vi "emi_Set Time offset.vi"(7 "Offset in":dbl, 11 "error in (no error)":errorcluster) -> (15 "error out":errorcluster)   [LabVIEW 2010]
doc: "Sets the get time with error and offset offset. Does not set teh clock, and does not store the time on disk.\n\nOn error, asume that the offset is wrong. Do nothing"
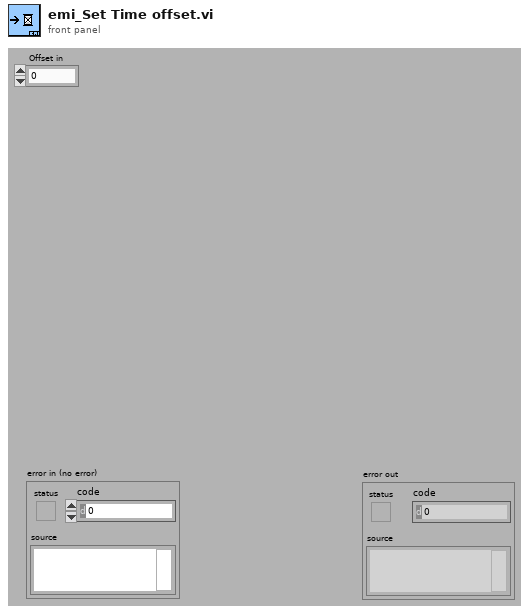
[diagram p1: front panel]
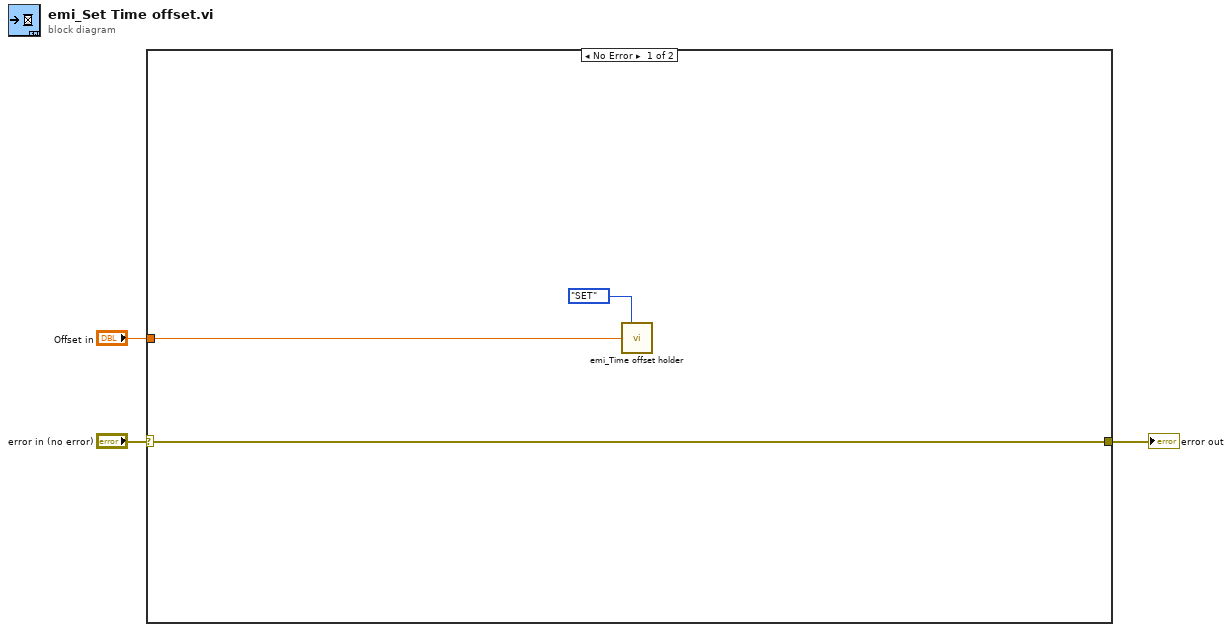
[diagram p0: block diagram]
diagram:
  n1 = case shown="No Error" "error in (no error)" {
    selector: "error in (no error)" -> [w6 w7]
    tunnel: [w6 w7] -> w2
    tunnel: "Offset in" -> [w5 _]
    frame No Error {
      n2 = call "emi_Time offset holder.vi"("Action(GET)"=enum16{"GET", "SET"}."SET", "Offset in"=w5) -> ()  [unwired: 13 in, 1 out]
    }
    frame Error {
    }
  }
  "error out" <- w2
